vi "Display Another Module VI--helper.vi"(8 "error in (no error)":errorcluster, 9 "Display Scenario":T1, 10 "Module DQMH Path":path) -> (0 "error out":errorcluster, 3 "Accept?":bool)   [LabVIEW 2020, in "UI Manager.lvlib"]
doc: "____\nHAMPEL SOFTWARE ENGINEERING v2.6.0 (2023-12-19 10:54)"
uses:
  UI Manager.lvlib
  Module Display Scenarios.ctl
  Libraries/hse-libraries/Source/hse-dqmh/hse-dqmh-dynamicrequesters.lvlib
  Libraries/hse-libraries/Source/hse-dqmh/hse-dqmh.lvlib
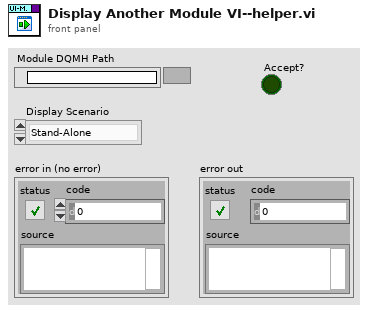
[diagram p1: front panel]
types:
  T1 = typedef "UI Manager.lvlib/Module Display Scenarios.ctl" = enum16{"Stand-Alone", "Managed"}
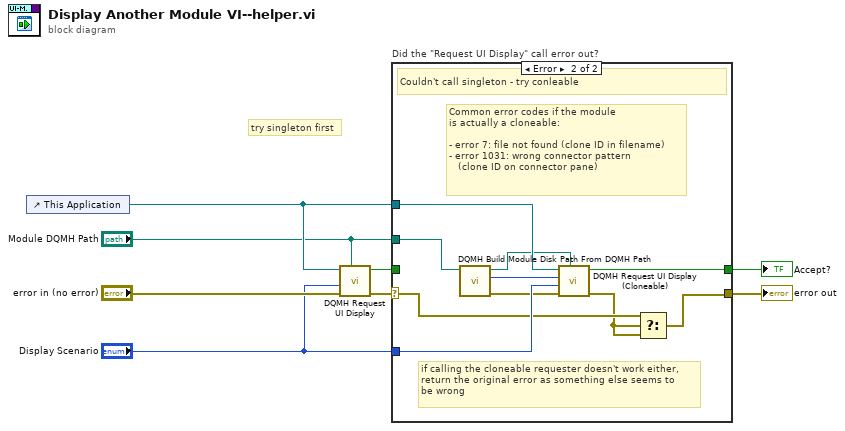
[diagram p0: block diagram]
diagram:
  # "try singleton first"
  n1 = control-ref of="This Application"() -> (w6:refnum<vi>)
  n2 = call "DQMH Request UI Display.vi"("Module DIsk Path"="Module DQMH Path", "error in (no error)"="error in (no error)", "Display Scenario"="Display Scenario", "Application reference"=w6) -> ("error out"=w7:errorcluster, "Accept?"=w3:bool)  [unwired: 6 in]
  n3 = case "Did the \"Request UI Display\" call error out?" shown="Error" w7 {
    selector: w7 -> [w9 w13]
    tunnel: "Module DQMH Path" -> [_ w19]
    tunnel: w6 -> [_ w20]
    tunnel: "Display Scenario" -> [_ w17]
    tunnel: [w9 w11] -> w4
    tunnel: [w10 w18] -> w2
    tunnel: w3 -> [w10 _]
    frame No Error {
    }
    frame Error {
      # "Common error codes if the module \nis actually a cloneable:\n\n- error 7: file not found (clone ID in filename)\n- error 1031: wrong connector pattern \n   (clone ID on connector pane)"
      # "if calling the cloneable requester doesn't work either,\nreturn the original error as something else seems to \nbe wrong"
      # "Couldn't call singleton - try conleable"
      n4 = call "DQMH Build Module Disk Path From DQMH Path.vi"("Module DQMH Path"=w19) -> ("error out"=w14:errorcluster, "Clone ID"=w16:i32, "Module Disk Path"=w15:path)  [unwired: 7 in, 1 out]
      n5 = call "DQMH Request UI Display (Cloneable).vi"("Module Disk Path"=w15, "error in (no error)"=w14, "Display Scenario"=w17, "Module ID"=w16, "Application reference"=w20) -> ("error out"=w12:errorcluster, "Accept?"=w18:bool)  [unwired: 5 in]
      n6 = Select(t=w13, s=w12, f=w12) -> (s? t:f=w11:errorcluster)
    }
  }
  "error out" <- w4
  "Accept?" <- w2
